vi "SetClimberSpeed.vi"(8 "error in":errorcluster, 11 "ClimberSpeed":dbl) -> (0 "error out":errorcluster)   [LabVIEW 2016]
uses:
  Robot Global Data.vi
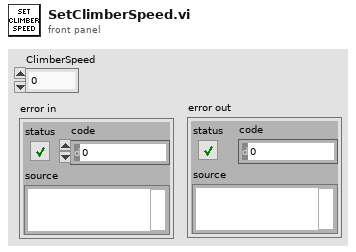
[diagram p1: front panel]
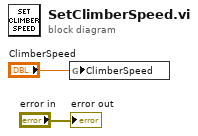
[diagram p0: block diagram]
diagram:
  n1 = global write "Robot Global Data.vi" "ClimberSpeed"("ClimberSpeed") -> ()
  "error out" <- "error in"
